vi "Zad1.vi"() -> ()   [LabVIEW 2017]
uses:
  <vilib>/measure/NI_MABase.lvlib
panel:
  out "input 2":dbl=10.0 format="%0.2p"
  in  "input":dbl=10.0 format="%0.2p"
  in  "frequency":dbl=10.0 format="%0.2p"
  out "Waveform Graph 2":waveform(dbl)(graph)
  out "Waveform Graph":waveform(dbl)(graph)
  in  "stop":bool
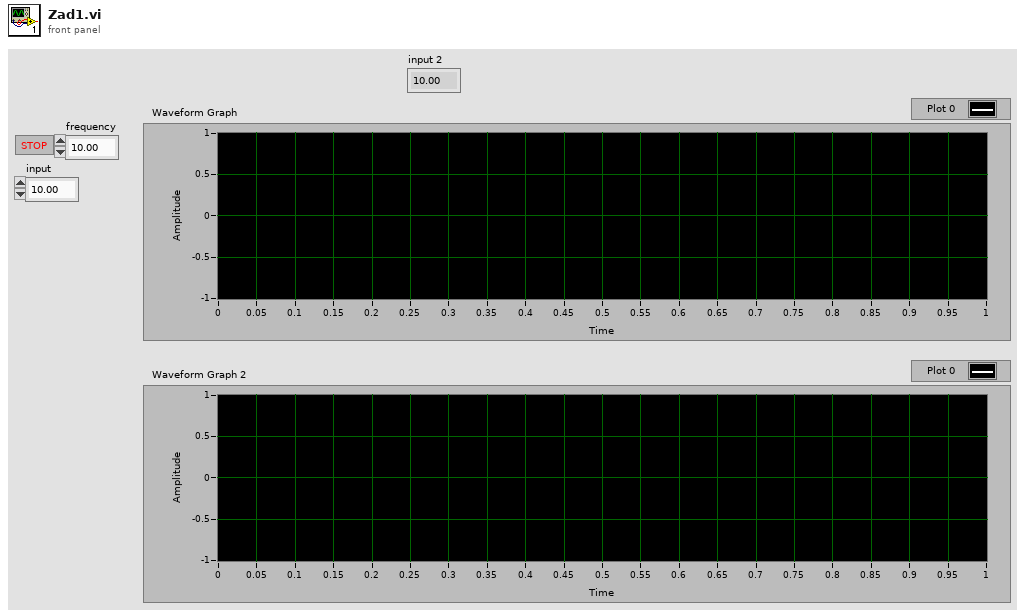
[diagram p1: front panel]
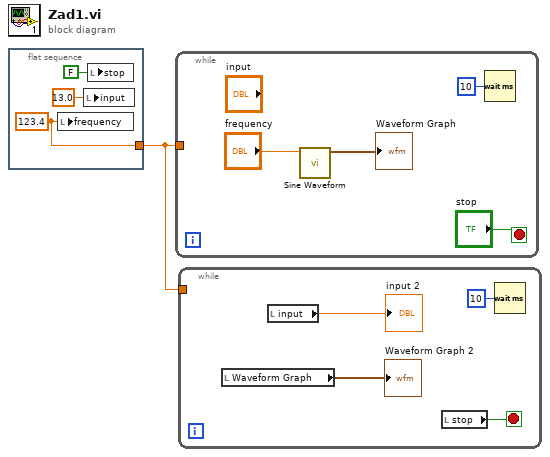
[diagram p0: block diagram]
diagram:
  n1 = flat-sequence {
    tunnel: [w2] -> w1
    frame #0 {
      w2 = 123.4 ("frequency")
      n2 = local write "frequency"(w2) -> ()
      n3 = local write "input"(13.0 ("input")) -> ()
      n4 = local write "stop"(FALSE ("stop")) -> ()
    }
  }
  n5 = while {
    tunnel: w1 -> [_]
    stop <- "stop" stop-if-true
    n6 = call <vilib>:"Sine Waveform.vi"("frequency"="frequency") -> ("signal out"=→"Waveform Graph":waveform(dbl))  [unwired: 9 in, 1 out]
    n7 = Wait (ms)(milliseconds to wait=u32 10) -> ()  [unwired: 1 out]
  }
  n8 = while {
    tunnel: w1 -> [_]
    stop <- w9 stop-if-true
    n9 = local read "Waveform Graph"() -> (→"Waveform Graph 2":waveform(dbl))
    n10 = local read "input"() -> (→"input 2":dbl)
    n11 = local read "stop"() -> (w9:bool)
    n12 = Wait (ms)(milliseconds to wait=u32 10) -> ()  [unwired: 1 out]
  }
